vi "Subvi buffer pixelclock.vi"   [LabVIEW 2017]
uses:
  <vilib>/rvi/Emulation/niFpgaSctlEmulationGetInTimedLoop.vi
  GV FIFOIN timeout.vi
  <vilib>/rvi/interface/RandomDataEmulation/niFpgaRandomDataHandleErrors.vi
  GV N pixelclock per line.vi
  <vilib>/rvi/Emulation/niFpgaProcessEmulError.vi
  <vilib>/rvi/Memory/Memory_Emulation/nirvimemoryFastEmulation.vi
  <vilib>/rvi/Memory/Memory_Emulation/nirvimemoryEmulation.vi
  <vilib>/rvi/Emulation/niFpgaEmulationIsFPGAContextNoSignature.vi
  <vilib>/rvi/DataTransferAndStorage/Container/Common/niFpgaContainerGetUniqueNameForEmu.vi
  <vilib>/rvi/errors/nirviReportUnexpectedCaseInternalError (U32).vi
  <vilib>/rvi/DataTransferAndStorage/Container/XNode/niFpgaContainer.xnode
  <vilib>/rvi/interface/RandomDataEmulation/nirviRandomDataFpgaReadWriteTemplate.vi
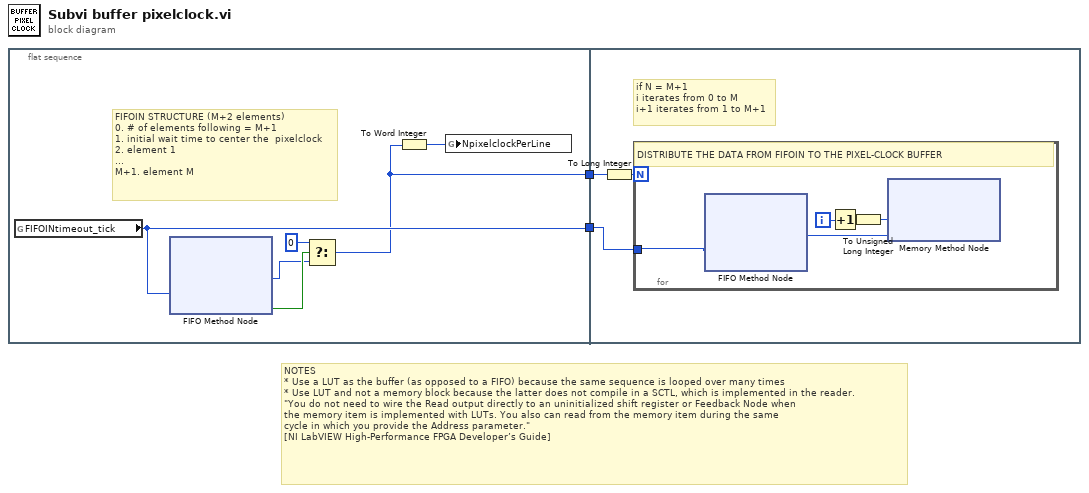
[diagram p0: block diagram]
diagram:
  # "NOTES\n* Use a LUT as the buffer (as opposed to a FIFO) because the same sequence is looped over many times\n* Use LUT and not a memory block because the latter does not compile in a SCTL, which is implemented in the reader.\n\"You do not need to wire the Read output directly to an uninitialized shift register or Feedback Node when\nthe memory item is implemented with LUTs. You also can read from the memory item during the same\ncycle in which you provide the Address parameter.\"\n[NI LabVIEW High-Performance FPGA Developer’s Guide]"
  n1 = flat-sequence {
    tunnel: [w7] -> w2
    tunnel: [w3] -> w1
    tunnel: w2 -> [w9]
    tunnel: w1 -> [w10]
    frame #0 {
      # "FIFOIN STRUCTURE (M+2 elements)\n0. # of elements following = M+1\n1. initial wait time to center the  pixelclock\n2. element 1\n...\nM+1. element M"
      n2 = global read "GV FIFOIN timeout.vi" "FIFOINtimeout_tick"() -> (w7:i32)
      n3 = xnode ("FIFO Method Node")("Timeout"=w7) -> ("Element"=w5:u32, "Timed Out?"=w6:bool)  [unwired: 1 in, 1 out]
      n4 = Select(t=u32 0, s=w6, f=w5) -> (s? t:f=w3:u32)
      n5 = To Word Integer(number=w3) -> (16bit integer=w4:i16)
      n6 = global write "GV N pixelclock per line.vi" "NpixelclockPerLine"(w4) -> ()
    }
    frame #1 {
      # "if N = M+1\ni iterates from 0 to M\ni+1 iterates from 1 to M+1"
      n7 = To Long Integer(number=w10) -> (32bit integer=w11:i32)
      n8 = for {
        N: w11 -> [_]
        tunnel: w9 -> [w16]
        i -> [w15]
        # "DISTRIBUTE THE DATA FROM FIFOIN TO THE PIXEL-CLOCK BUFFER"
        n9 = xnode ("FIFO Method Node")("Timeout"=w16) -> ("Element"=w12:u32)  [unwired: 1 in, 2 out]
        n10 = Increment(x=w15) -> (x+1=w14:i32)
        n11 = To Unsigned Long Integer(number=w14) -> (unsigned 32bit integer=w13:u32)
        n12 = xnode ("Memory Method Node")("Address"=w13, "Data"=w12) -> ()  [unwired: 1 in, 1 out]
      }
    }
  }
